vi "New FPGATarget.vi"(8 "instVIpath":path, 9 "target location":string, 11 "FPGAtarget in":refnum<class "FPGATarget.lvclass">) -> (3 "FPGAtarget out":refnum<class "FPGATarget.lvclass">)   [LabVIEW 2020, in "NI_TargetHelper.lvlib" / "FPGATarget.lvclass"]
uses:
  <vilib>/TargetSupport/NI_TargetHelper/FPGATarget/FPGATarget.lvclass
  <vilib>/TargetSupport/NI_TargetHelper/FPGATarget/FPGATarget.lvclass/FPGATarget.ctl
  <vilib>/TargetSupport/NI_TargetHelper/NI_TargetHelper.lvlib
panel:
  out "error out":errorcluster
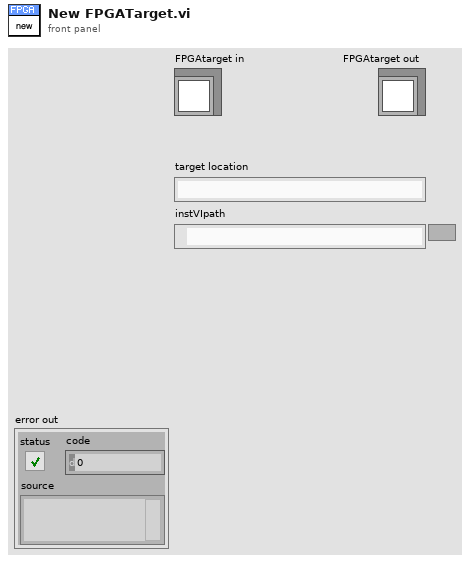
[diagram p1: front panel]
types:
  T1 = typedef "NI_TargetHelper.lvlib/Instance VIref.ctl" = refnum<vi>
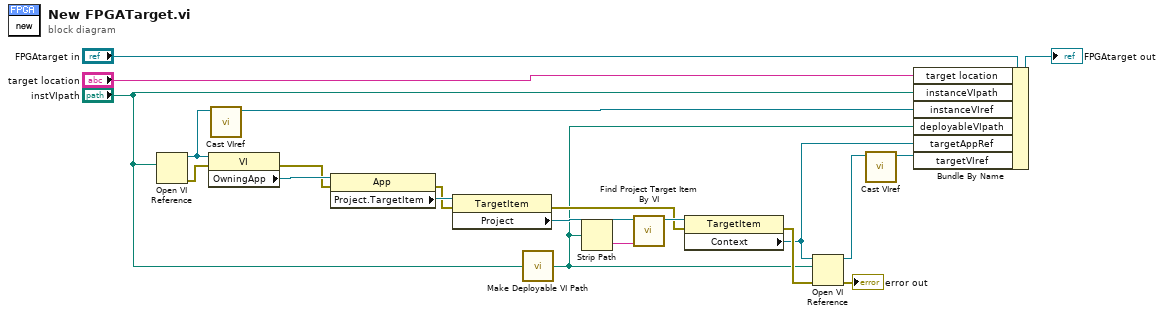
[diagram p0: block diagram]
diagram:
  n1 = Open VI Reference(vi path="instVIpath") -> (vi reference=w7:refnum<vi>, error out=w13:errorcluster)  [unwired: 5 in]
  n2 = property class="VI"(reference=w7, error in=w13) -> (error out=w12:errorcluster, "OwningApp"=w17:refnum<vi>)  [unwired: 1 out]
  n3 = call <vilib>:"Cast VIref.vi"("VI Refnum"=w7) -> ("instVIref"=w4:T1)  [unwired: 10 in]
  n4 = property class="App"(reference=w17, error in=w12) -> (error out=w11:errorcluster, "Project.TargetItem"=w18:refnum<vi>)  [unwired: 1 out]
  n5 = property class="TargetItem"(reference=w18, error in=w11) -> (error out=w10:errorcluster, "Project"=w16:refnum<vi>)  [unwired: 1 out]
  n6 = call <vilib>:"Make Deployable VI Path.vi"("instance path"="instVIpath") -> ("deployable path"=w3:path)
  n7 = Strip Path(path=w3) -> (name=w19:string)  [unwired: 1 out]
  n8 = call <vilib>:"Find Project Target Item By VI.vi"("vi name"=w19, "project"=w16) -> ("TargetItem Refnum"=w15:refnum<vi>)  [unwired: 8 in, 1 out]
  n9 = property class="TargetItem"(reference=w15, error in=w10) -> (error out=w9:errorcluster, "Context"=w2:refnum<vi>)  [unwired: 1 out]
  n10 = Open VI Reference(application reference (local)=w2, vi path=w3, error in (no error)=w9) -> (vi reference=w14:refnum<vi>, error out=→"error out":errorcluster)  [unwired: 3 in]
  n11 = call <vilib>:"Cast VIref.vi"("VI Refnum"=w14) -> ("instVIref"=w1:T1)  [unwired: 10 in]
  n12 = Bundle By Name(cluster="FPGAtarget in", "target location"="target location", "instanceVIpath"="instVIpath", "instanceVIref"=w4, "deployableVIpath"=w3, "targetAppRef"=w2, "targetVIref"=w1) -> (→"FPGAtarget out":refnum<class "FPGATarget.lvclass">)
